vi "Write Output_Enable.vi"(8 "error in":errorcluster, 10 "Output_Enable":bool, 11 "36234A in":refnum<class "36234A.lvclass">) -> (0 "error out":errorcluster, 3 "36234A out":refnum<class "36234A.lvclass">)   [LabVIEW 2019, in "36234A.lvlib" / "36234A.lvclass"]
uses:
  Library/36234A.lvclass
  C:/Users/Public/Documents/Development/builds/Instruments/PowerSupply.lvlibp/Library/PowerSupply.lvclass
  Library/36234A.lvclass/36234A.ctl
  builds/Instruments/PowerSupply.lvlibp/Accessors/Read Active Channel.vi
  builds/Instruments/PowerSupply.lvlibp/Library/PowerSupply.lvclass
  <instrlib>/Keysight E36000 Series/Keysight E36000 Series.lvlib
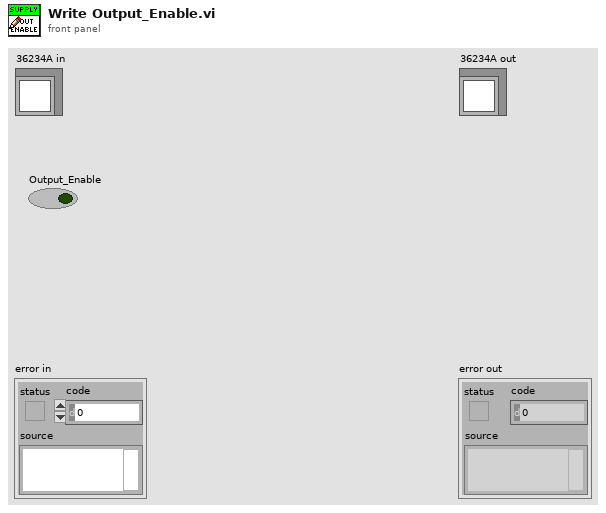
[diagram p1: front panel]
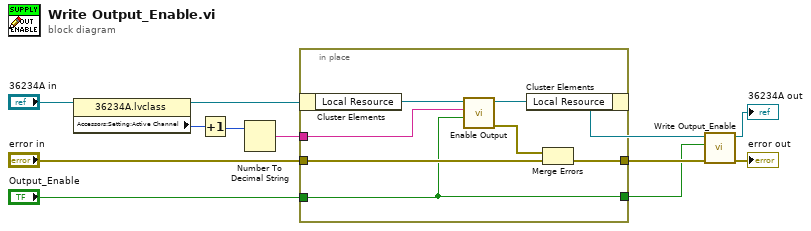
[diagram p0: block diagram]
diagram:
  n1 = property class="36234A.lvclass"(reference="36234A in") -> (reference out=w7:refnum<class "36234A.lvclass">, "Accessors:Setting:Active Channel"=w6:u32)  [unwired: 1 in, 1 out]
  n2 = Increment(x=w6) -> (x+1=w5:u32)
  n3 = Number To Decimal String(number=w5) -> (decimal integer string=w4:string)  [unwired: 1 in]
  n4 = in-place {
    in-place-border: "error in" -> [w16]
    in-place-border: w4 -> [w17]
    in-place-border: [w14] -> w3
    in-place-border: "Output_Enable" -> [w13]
    in-place-border: [w13] -> w1
    n5 = in-place-cluster #1(w7) -> ("Local Resource"=w19:refnum<visa-resource-name>)
    n6 = call <instrlib>:"Enable Output.vi"("Enable Output (F: Disable)"=w13, "Channel (1)"=w17, "VISA resource name"=w19) -> ("error out"=w15:errorcluster, "VISA resource name out"=w18:refnum<visa-resource-name>)  [unwired: 7 in]
    n7 = in-place-cluster #1("Local Resource"=w18) -> (w10:refnum<class "36234A.lvclass">)
    n8 = Merge Errors(w15, w16) -> (w14:errorcluster)
  }
  n9 = call-parent "Write Output_Enable.vi"("error in"=w3, "Output_Enable"=w1, "PowerSupply in"=w10) -> ("error out"=→"error out":errorcluster, "PowerSupply out"=→"36234A out":refnum<class "36234A.lvclass">)  [unwired: 7 in]
